vi "InsertItem2XMenu.vi"(8 "error in (no error)":errorcluster, 9 "Item":T1, 10 "InserAfterTag":string, 11 "CMenu in":refnum<class "CMenu.lvclass">) -> (0 "error out":errorcluster, 3 "CMenu out":refnum<class "CMenu.lvclass">)   [LabVIEW 2009]
doc: "Insert a Item to the menu database"
uses:
  CMenu.lvclass
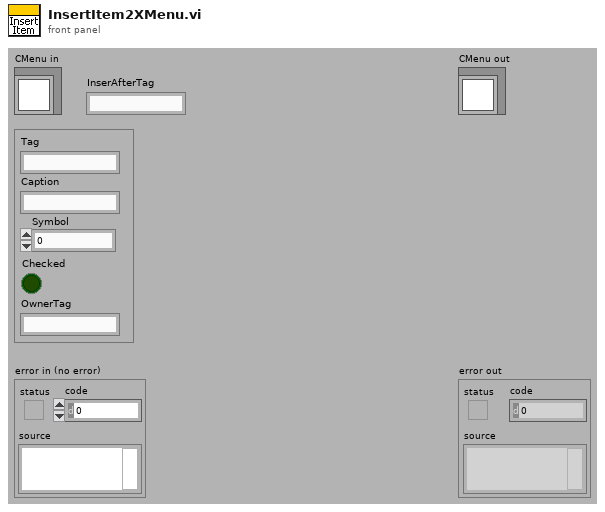
[diagram p1: front panel]
types:
  T1 = cluster{"Tag":string, "Caption":string, "Symbol":i32, "Checked":bool, "OwnerTag":string}
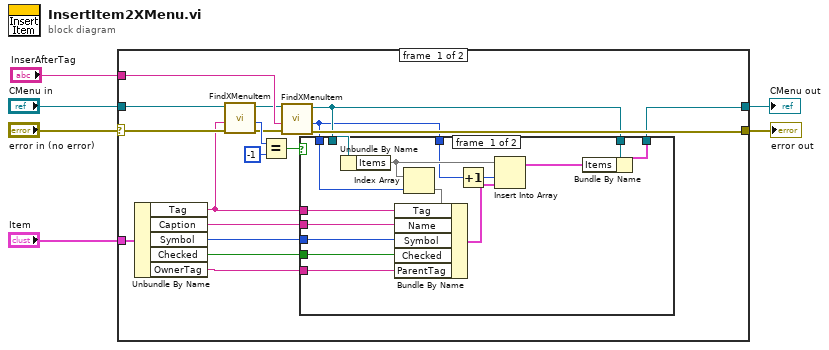
[diagram p0: block diagram]
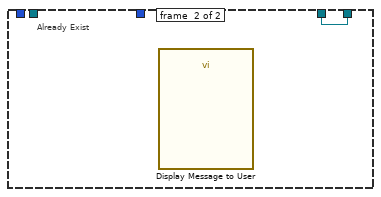
[diagram p2: hidden frame]
diagram:
  n1 = case shown="No Error" "error in (no error)" {
    selector: "error in (no error)" -> [w18 w42]
    tunnel: [w16 w42] -> w5
    tunnel: [w7 w41] -> w3
    tunnel: "CMenu in" -> [w19 w41]
    tunnel: "Item" -> [w24 _]
    tunnel: "InserAfterTag" -> [w23 _]
    frame #0 {
      n2 = Unbundle By Name(w24) -> ("Tag"=w13:string, "Caption"=w12:string, "Symbol"=w11:i32, "Checked"=w10:bool, "OwnerTag"=w9:string)
      n3 = call "FindXMenuItem.vi"("error in (no error)"=w18, "ItemTag"=w13, "CMenu in"=w19) -> ("error out"=w17:errorcluster, "Index"=w22:i32, "CMenu out"=w15:refnum<class "CMenu.lvclass">)  [unwired: 6 in]
      n4 = Equal?(x=w22, y=-1) -> (x = y?=w20:bool)
      n5 = call "FindXMenuItem.vi"("error in (no error)"=w17, "ItemTag"=w23, "CMenu in"=w15) -> ("error out"=w16:errorcluster, "Index"=w8:i32, "CMenu out"=w14:refnum<class "CMenu.lvclass">)  [unwired: 6 in]
      n6 = case shown="False" w20 {
        tunnel: w14 -> [w39 _]
        tunnel: w8 -> [w28 _]
        tunnel: w14 -> [w35 w40]
        tunnel: [w33 w40] -> w7
        tunnel: w13 -> [w32 _]
        tunnel: w12 -> [w31 _]
        tunnel: w11 -> [w30 _]
        tunnel: w10 -> [w29 _]
        tunnel: w9 -> [w25 _]
        tunnel: w8 -> [w27 _]
        frame #0 {
          n7 = Unbundle By Name(w39) -> ("Items"=w38)
          n8 = Index Array(array=w38, index=w28) -> (element=w37)
          n9 = Bundle By Name(cluster=w37, "Tag"=w32, "Name"=w31, "Symbol"=w30, "Checked"=w29, "ParentTag"=w25) -> (w36:cluster{})
          n10 = Increment(x=w27) -> (x+1=w26:i32)
          n11 = Insert Into Array(array=w38, index=w26, new element=w36) -> (w34:cluster{}[])
          n12 = Bundle By Name(cluster=w35, "Items"=w34) -> (w33:cluster{})
        }
        frame #1 {
          # "Already Exist"
          n13 = call "Display Message to User"() -> ()  [unwired: 10 in, 2 out]
        }
      }
    }
    frame #1 {
    }
  }
  "error out" <- w5
  "CMenu out" <- w3
